vi "endianSwitch.vi"(11 "U16 array in":u16[](array[numeric])) -> (3 "U16 array out":u16[](array[numeric]))   [LabVIEW 2020]
doc: "Exchange odd-indexed and even-indexed elements in <B>U16 array in</B>."
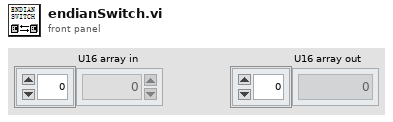
[diagram p1: front panel]
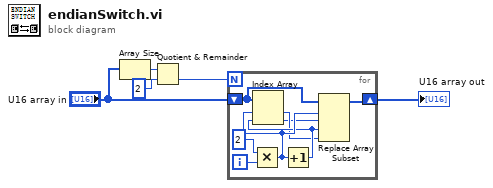
[diagram p0: block diagram]
diagram:
  n1 = Array Size(array="U16 array in") -> (size(s)=w3:i32)
  n2 = Quotient & Remainder(x=w3, y=2) -> (floor(x/y)=w1:i32)  [unwired: 1 out]
  n3 = for {
    N: w1 -> [_]
    shift-right: [w6] -> w5
    shift-left: "U16 array in" -> [w11]
    i -> [w13]
    n4 = Multiply(x=2, y=w13) -> (x*y=w10:i32)
    n5 = Increment(x=w10) -> (x+1=w9:i32)
    n6 = Index Array(array=w11, index #1=w10, index #2=w9) -> (element #1=w8:u16, element #2=w7:u16)
    n7 = Replace Array Subset(array=w11, new element #1=w7, index #1=w10, new element #2=w8, index #2=w9) -> (w6:u16[])
  }
  "U16 array out" <- w5
